vi "QueuedStateMachine.vi"() -> ()   [LabVIEW 2020]
panel:
  in  "State":T1(ring)=enum."Idle"
  out "error out":errorcluster
  in  "error in":errorcluster
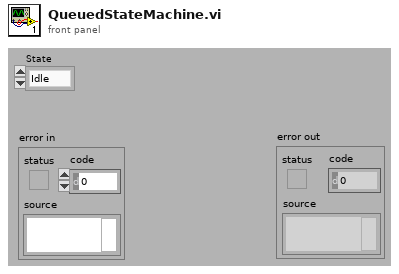
[diagram p1: front panel]
types:
  T1 = enum16{"Initialize", "Idle", "State1", "State2", "State3", "STOP"}
  T2 = enum16{"Initialize", "Idle", "State1", "State2", "State3", "STOP"}[]
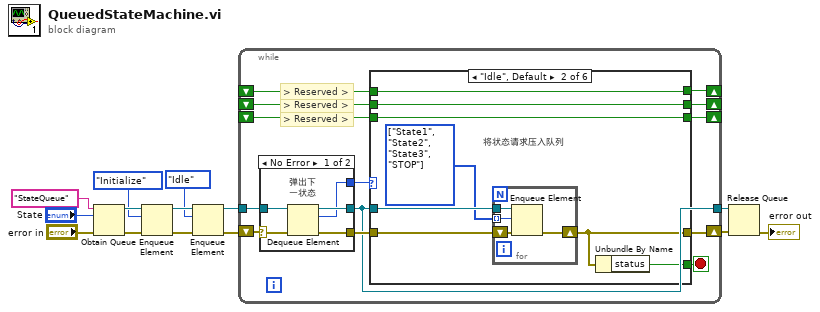
[diagram p0: block diagram]
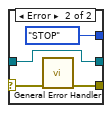
[diagram p2: hidden frame]
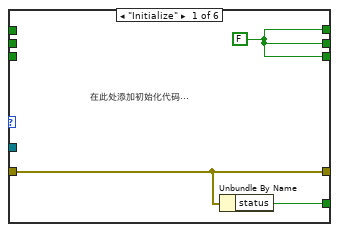
[diagram p3: hidden frame]
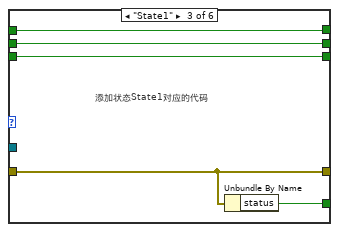
[diagram p4: hidden frame]
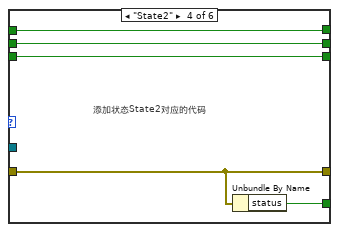
[diagram p5: hidden frame]
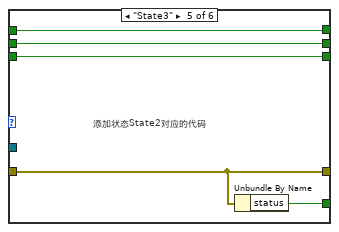
[diagram p6: hidden frame]
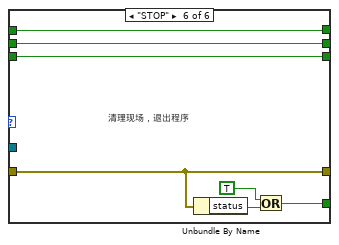
[diagram p7: hidden frame]
diagram:
  n1 = Obtain Queue(name (unnamed)="StateQueue", element data type="State", error in (no error)="error in") -> (queue out=w13:refnum<queue>, error out=w12:errorcluster)  [unwired: 2 in, 1 out]
  n2 = Enqueue Element(queue=w13, element=T1."Initialize", error in (no error)=w12) -> (queue out=w6:refnum<queue>, error out=w7:errorcluster)  [unwired: 1 in, 1 out]
  n3 = Enqueue Element(queue=w6, element=T1."Idle", error in (no error)=w7) -> (queue out=w5:refnum<queue>, error out=w4:errorcluster)  [unwired: 1 in, 1 out]
  n4 = while {
    shift-right: [w26] -> w11
    shift-left: w4 -> [w18]
    shift-right: [w22] -> _
    shift-left: _ -> [w20]
    shift-right: [w25] -> _
    shift-left: _ -> [w23]
    shift-right: [w24] -> _
    shift-left: _ -> [w21]
    tunnel: w5 -> [w19]
    tunnel: [w16] -> w10
    stop <- w27 stop-if-true
    # "> Reserved >"
    # "> Reserved >"
    # "> Reserved >"
    n5 = case shown="No Error" w18 {
      selector: w18 -> [w31 w36]
      tunnel: w19 -> [w32 w35]
      tunnel: [w30 w35] -> w16
      tunnel: [w29 w34] -> w17
      tunnel: [w28 T1."STOP"] -> w15
      frame No Error {
        # "弹出下\n一状态"
        n6 = Dequeue Element(queue=w32, error in (no error)=w31) -> (queue out=w30:refnum<queue>, element=w28:T1, error out=w29:errorcluster)  [unwired: 1 in, 1 out]
      }
      frame Error {
        n7 = call <vilib>:"General Error Handler.vi"("error in (no error)"=w36) -> ("error out"=w34:errorcluster)  [unwired: 10 in, 4 out]
      }
    }
    n8 = case shown="\"Idle\", Default" w15 {
      tunnel: [w38 w43 w52 w57 w62 w69] -> w27
      tunnel: w17 -> [w37 w47 w53 w58 w63 w70]
      tunnel: [w37 w44 w53 w58 w63 w70] -> w26
      tunnel: [w39 w41 w55 w60 w64 w72] -> w25
      tunnel: [w39 w40 w56 w59 w65 w71] -> w24
      tunnel: w23 -> [_ w41 w55 w60 w64 w72]
      tunnel: [w39 w42 w54 w61 w66 w73] -> w22
      tunnel: w21 -> [_ w40 w56 w59 w65 w71]
      tunnel: w20 -> [_ w42 w54 w61 w66 w73]
      tunnel: w16 -> [_ w46 _ _ _ _]
      frame "Initialize" {
        w39 = FALSE
        # "在此处添加初始化代码..."
        n9 = Unbundle By Name(w37) -> ("status"=w38:bool)
      }
      frame "Idle", Default {
        w45 = T2 [enum."State1", enum."State2", enum."State3", enum."STOP"] items=["Initialize", "Idle", "State1", "State2", "State3", "STOP"]
        # "将状态请求压入队列"
        n10 = for {
          tunnel: w46 -> [w49]
          shift-right: [w50] -> w44
          shift-left: w47 -> [w51]
          tunnel: w45 -> [w48] mode=indexing
          n11 = Enqueue Element(queue=w49, element=w48, error in (no error)=w51) -> (error out=w50:errorcluster)  [unwired: 1 in, 2 out]
        }
        n12 = Unbundle By Name(w44) -> ("status"=w43:bool)
      }
      frame "State1" {
        # "添加状态State1对应的代码"
        n13 = Unbundle By Name(w53) -> ("status"=w52:bool)
      }
      frame "State2" {
        # "添加状态State2对应的代码"
        n14 = Unbundle By Name(w58) -> ("status"=w57:bool)
      }
      frame "State3" {
        # "添加状态State2对应的代码"
        n15 = Unbundle By Name(w63) -> ("status"=w62:bool)
      }
      frame "STOP" {
        # "清理现场，退出程序"
        n16 = Unbundle By Name(w70) -> ("status"=w68:bool)
        n17 = Or(x=TRUE, y=w68) -> (x .or. y?=w69:bool)
      }
    }
  }
  n18 = Release Queue(queue=w10, error in (no error)=w11) -> (error out=→"error out":errorcluster)  [unwired: 1 in, 2 out]
